vi "SensorInterrupt.vi"(8 "error in (no error)":errorcluster, 11 "CubeLift in":refnum<class "CubeLift.lvclass">) -> (0 "error out":errorcluster, 3 "CubeLift out":refnum<class "CubeLift.lvclass">)   [LabVIEW 2017, in "CubeLift.lvclass"]
uses:
  CubeLift.lvclass
  Subsystem.lvclass
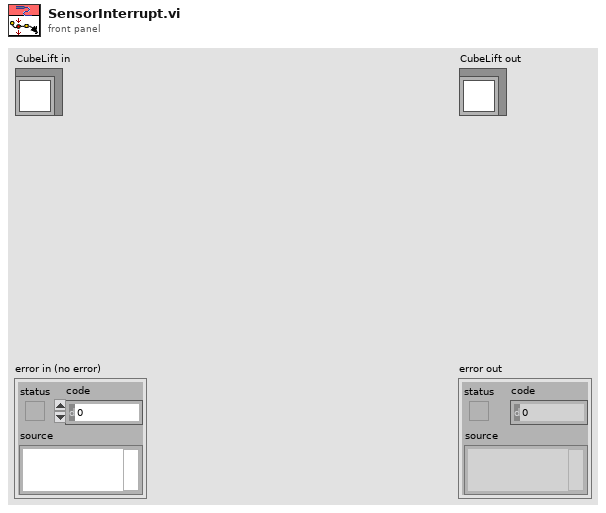
[diagram p1: front panel]
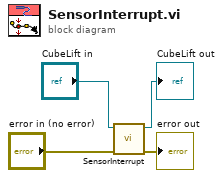
[diagram p0: block diagram]
diagram:
  n1 = call-parent "SensorInterrupt.vi"("error in (no error)"="error in (no error)", "Subsystem in"="CubeLift in") -> ("error out"=→"error out":errorcluster, "Subsystem out"=→"CubeLift out":refnum<class "CubeLift.lvclass">)  [unwired: 8 in]
